vi "LcWebView_BarPlot_Example.vi"() -> ()   [LabVIEW 2019, in "LcWebView.lvclass"]
doc: "Inject javascript arguments"
uses:
  LcWebView.lvclass
  ctrls/PlotType.ctl
  ctrls/BarPlotOption.ctl
  Program Files/National Instruments/LabVIEW 2020/user.lib/_LabVIEWCommon/LcHTMLPlot/HTMLPlot_class/Controls/LegendPosition.ctl
  Program Files/National Instruments/LabVIEW 2020/user.lib/_LabVIEWCommon/LcHTMLPlot/HTMLPlot_class/HTMLPlot.lvclass
  ctrls/GenericPlotOption.ctl
  C:/Projects/WebView2/LcWebView/data/Microsoft.Web.WebView2.WinForms.dll
panel:
  out "BrowserProcessId":u32
  out "Source Change":string
  out "Status Message":string
  in  "stop":bool
  in  "Web":refnum<k24>(container)
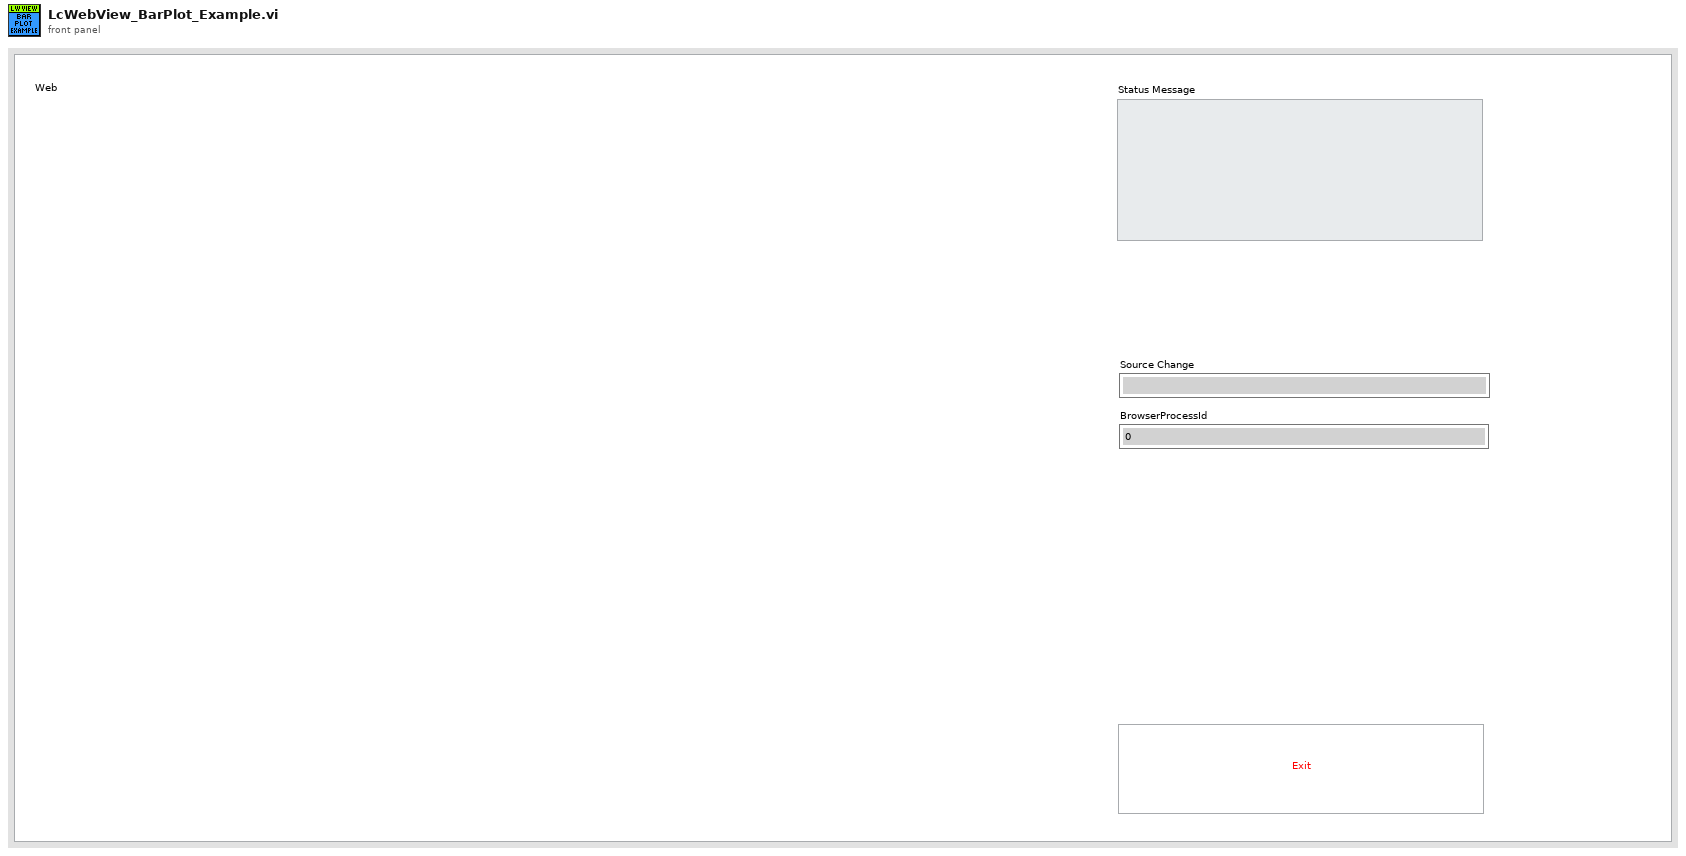
[diagram p1: front panel]
types:
  T1 = typedef "LcWebView.lvclass/PlotType.ctl" = enum16{"bar", "line", "pie"}
  T2 = typedef "LcWebView.lvclass/GenericPlotOption.ctl" = cluster{"GraphTitle":string, "LegendDisplay":bool, "LegendPosition":T3}
  T3 = typedef "HTMLPlot.lvclass/LegendPosition.ctl" = enum16{"top", "right", "left", "bottom"}
  T4 = typedef "LcWebView.lvclass/BarPlotOption.ctl" = cluster{"xLabel":string, "yLabel":string, "DisplayXLabel":bool, "DisplayYLabel":bool, "Stacked":bool}
  T5 = typedef "LcWebView.lvclass/WebViewDynamicEvents.ctl" = cluster{"Event Registration Ref":refnum<event-registration>, "Source event":refnum<user-event>}
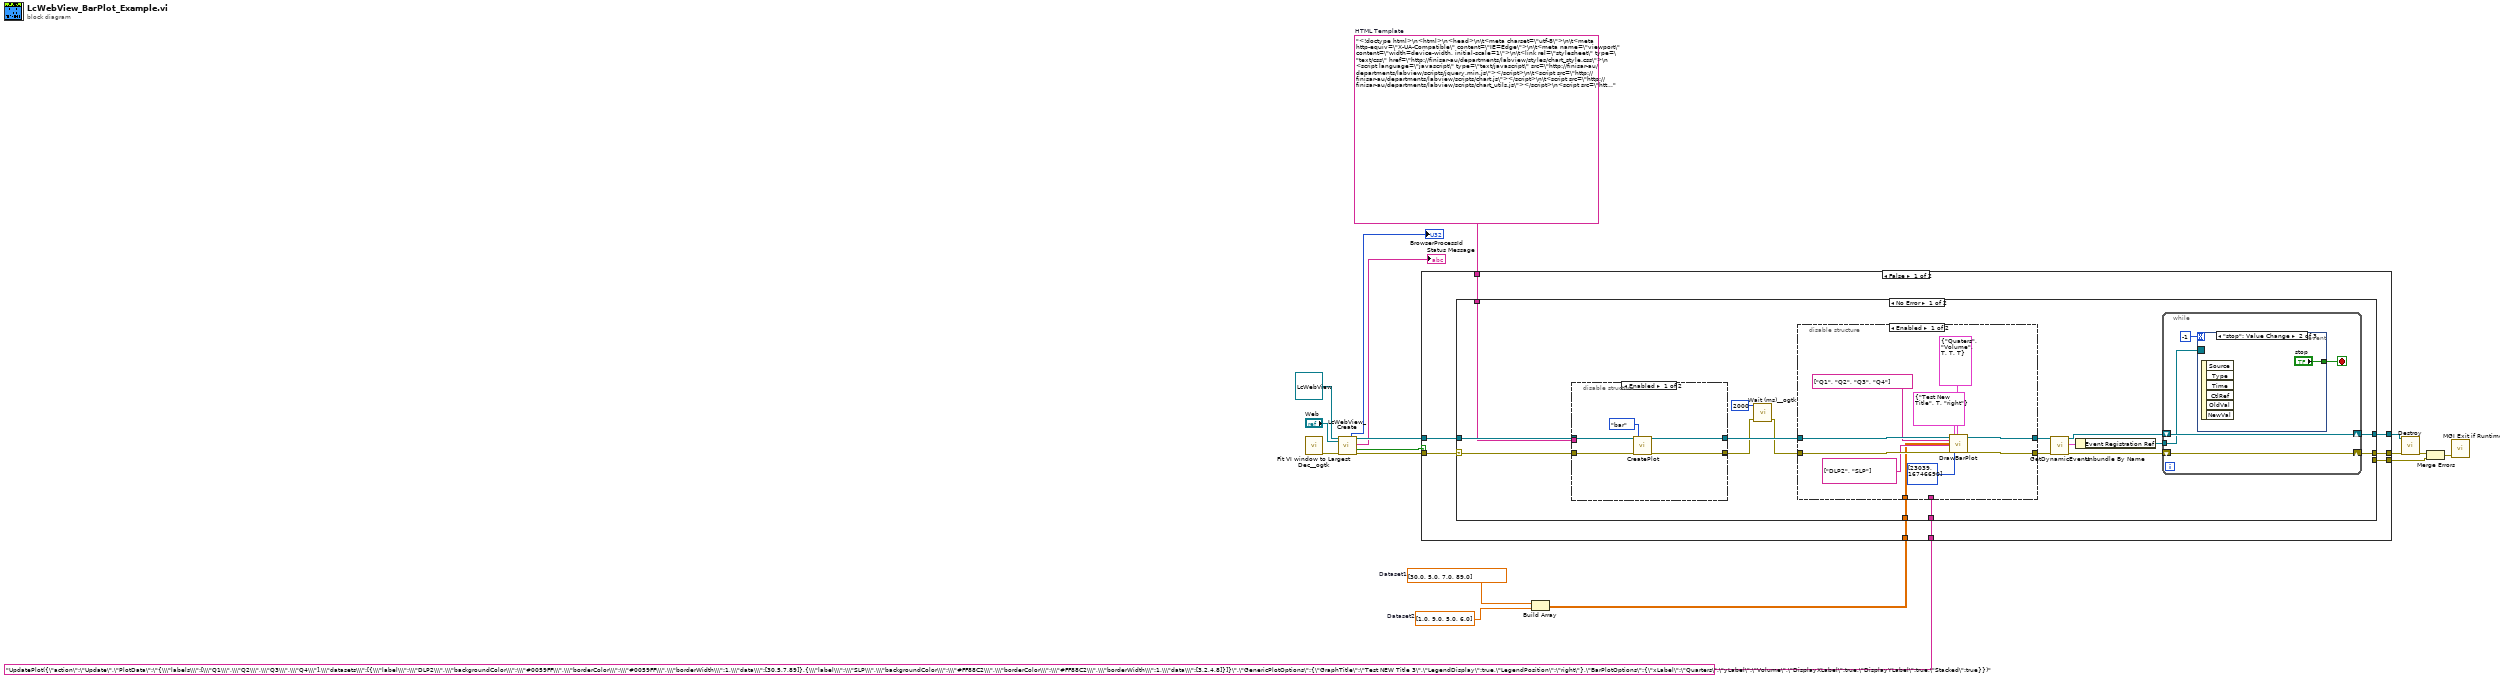
[diagram p0: block diagram]
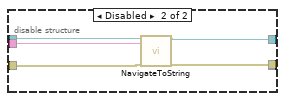
[diagram p2: hidden frame]
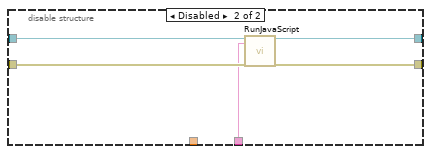
[diagram p3: hidden frame]
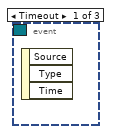
[diagram p4: hidden frame]
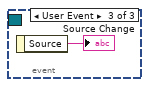
[diagram p5: hidden frame]
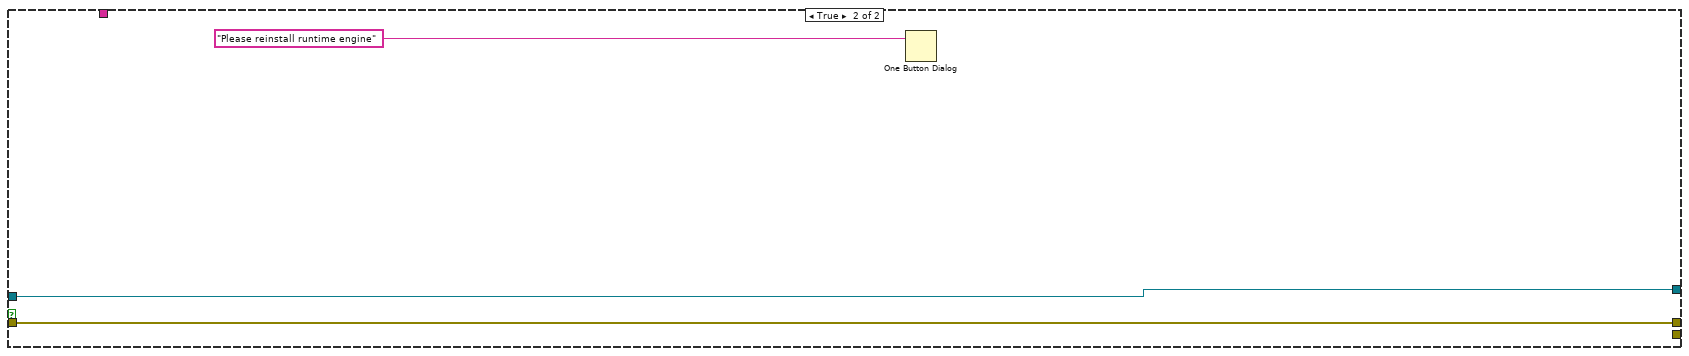
[diagram p7: hidden frame]
diagram:
  w1 = "<!doctype html>\n<html>\n<head>\n\t<meta charset=\"utf-8\">\n\t<meta http-equiv=\"X-UA-Compatible\" content=\"IE=Edge\">\n\t<meta name=\"viewport\" content=\"width=device-width, initial-scale=1\">\n\t<link rel=\"stylesheet\" type=\"text/css\" href=\"http://finisar-au/departments/labview/styles/chart_style.css\">\n <script language=\"javascript\" type=\"text/javascript\" src=\"http://finisar-au/departments/labview/scripts/jquery.min.js\"></script>\n\t<script src=\"http://finisar-au/departments/labview/scripts/chart.js\"></script>\n\t<script src=\"http://finisar-au/departments/labview/scripts/chart_utils.js\"></script>\n<script src=\"http://finisar-au/departments/labview/scripts/json2.js\"></script>\n    <script src=\"http://finisar-au/departments/labview/scripts/jquery(v1.11.3).min.js\"></script>\n    <style>\n    \t#container{\n            width:95vm;\n            height:95vh;\n            }\n        #canvas {\n\t\t-moz-user-select: none;\n\t\t-webkit-user-select: none;\n\t\t-ms-user-select: none;  \n\t   }\n\t    </style>\n</head>\n\n<body>\n<div id=\"container\">\n\t\t<canvas id=\"canvas\"></canvas>\n\t</div>\n\t<script type=\"text/javascript\">\n//---colour helper\nvar color = Chart.helpers.color;\nvar plotData ={}  \n\n // summarise config here --------------------------                   \n        var config = {\n\n// **************** PLOT TYPE***************************\n\t\t\ttype: 'bar',\n\n\t\t\tdata: plotData,\n//\t\t\t **************** PLOT OPTIONS : THIS PART WILL BE PLOT TYPE DEPENDENT***************************\noptions: \n{\nresponsive: true,\nmaintainAspectRatio: false,\n\t\t\t\tanimation: {\n\t\t\t\t\tanimateScale: true,\n\t\t\t\t\tanimateRotate: true\n\t\t\t\t},\nlegend: {\ndisplay:false,\t\t\t\t\t\t\nposition: 'right'\n\t\t\t\t\t},\ntitle: {\n\t\t\t\t\t\tdisplay:true,\n\t\t\t\t\t\ttext: 'INPUT'\n\t\t\t\t\t},  \n//*************************  ADDITIONAL OPTIONS   ***********************\n\t\t\t\tscales: {\n\t\t\t\t\txAxes: [{\n\t\t\t\t\t\t\tscaleLabel: {\n\t\t\t\t\t\t\tdisplay: true,\n\t\t\t\t\t\t\tlabelString: 'INPUT',\n       stacked:true\n\t\t\t\t\t\t}\n\t\t\t\t\t}],\n\t\t\t\t\tyAxes: [{\n\tticks: {\n\t\t\t\t\t\t\tmin: 0\n\t\t\t\t\t\t\t\t\t\t\t\t\t},\n\t\t\t\t\t\tscaleLabel: {\n\t\t\t\t\t\t\tdisplay: true,\n\t\t\t\t\t\t\tlabelString: 'INPUT',\n       stacked:true\n       \t\t\t\t\t\t}\n\t\t\t\t\t}]\n\t\t\t\t},\ntooltips: {\nenabled: true}\t\n}\n\t\t};\n\n// run plot function here -------------------------- \nwindow.onload = function() {\n\t  var ctx = document.getElementById('canvas').getContext('2d');\n\t\t\twindow.myChart = new Chart(ctx, config); \n};\n\nfunction UpdatePlot(data) {        \n    var myData = JSON.parse(data.PlotData);\n    config.data=myData;\n\tconfig.options.legend.display= data.GenericPlotOptions.LegendDisplay;\n\tconfig.options.legend.position=data.GenericPlotOptions.LegendPosition;            \n\tconfig.options.title.text=data.GenericPlotOptions.GraphTitle;\n\n//*************************  ADDITIONAL OPTIONS UPDATE ***********************\n\tconfig.options.scales.yAxes[0].stacked=data.BarPlotOptions.Stacked;\n\tconfig.options.scales.xAxes[0].stacked=data.BarPlotOptions.Stacked;\n\tconfig.options.scales.xAxes[0].scaleLabel.labelString=data.BarPlotOptions.xLabel;\n\tconfig.options.scales.yAxes[0].scaleLabel.labelString=data.BarPlotOptions.yLabel;\n\tconfig.options.scales.yAxes[0].scaleLabel.display=data.BarPlotOptions.DisplayYLabel;\n\tconfig.options.scales.xAxes[0].scaleLabel.display=data.BarPlotOptions.DisplayXLabel;\n\n//*************************  UPDATE PLOT ***********************\n\twindow.myChart.update();\n}\n\t</script>\n</body>\n</html>"  # HTML Template
  w5 = dbl[] [1.0, 9.0, 5.0, 6.0]  # Dataset2
  w4 = dbl[] [30.0, 5.0, 7.0, 89.0]  # Dataset1
  n1 = call "Fit VI window to Largest Dec__ogtk.vi"() -> ("error out"=w8:errorcluster)  [unwired: 6 in, 1 out]
  n2 = call "LcWebView_Create.vi"("reference in"=refnum<class "LcWebView.lvclass"> refnum, "Webview container"="Web", "Error In"=w8) -> ("BrowserProcessId"=→"BrowserProcessId":u32, "reference out"=w16:refnum<class "LcWebView.lvclass">, "Status Message"=→"Status Message":string, "Reinstall Runtime"=w9:bool, "Error Out"=w15:errorcluster)  [unwired: 9 in, 3 out]
  n3 = Build Array(w4, w5) -> (w3:dbl[][])
  n4 = case shown="False" w9 {
    tunnel: w16 -> [w26 w80]
    tunnel: w15 -> [w25 w79]
    tunnel: [w24 w80] -> w14
    tunnel: [w22 w79] -> w13
    tunnel: [w23 _] -> w10
    tunnel: w3 -> [w21 _]
    tunnel: "UpdatePlot({\"action\":\"Update\",\"PlotData\":\"{\\\"labels\\\":[\\\"Q1\\\",\\\"Q2\\\",\\\"Q3\\\",\\\"Q4\\\"],\\\"datasets\\\":[{\\\"label\\\":\\\"DLP2\\\",\\\"backgroundColor\\\":\\\"#0059FF\\\",\\\"borderColor\\\":\\\"#0059FF\\\",\\\"borderWidth\\\":1,\\\"data\\\":[30,5,7,89]},{\\\"label\\\":\\\"SLP\\\",\\\"backgroundColor\\\":\\\"#FF88C2\\\",\\\"borderColor\\\":\\\"#FF88C2\\\",\\\"borderWidth\\\":1,\\\"data\\\":[3,2,4,8]}]}\",\"GenericPlotOptions\":{\"GraphTitle\":\"Test NEW Title 3\",\"LegendDisplay\":true,\"LegendPosition\":\"right\"},\"BarPlotOptions\":{\"xLabel\":\"Quarters\",\"yLabel\":\"Volume\",\"DisplayXLabel\":true,\"DisplayYLabel\":true,\"Stacked\":true}})" ("Java Script Function") -> [w20 _]
    tunnel: w1 -> [w19 _]
    frame False {
      n5 = case shown="No Error" w25 {
        selector: w25 -> [w40 w76]
        tunnel: w26 -> [w41 w77]
        tunnel: [w37 w77] -> w24
        tunnel: [w43 _] -> w22
        tunnel: [_ w76] -> w23
        tunnel: w21 -> [w32 _]
        tunnel: w20 -> [w31 _]
        tunnel: w19 -> [w30 _]
        frame No Error {
          n6 = disable-structure shown="Enabled" {
            disable-tunnel: w41 -> [w48 w53]
            disable-tunnel: w40 -> [w47 w50]
            disable-tunnel: [w45 _] -> w29
            disable-tunnel: [w44 w52] -> w33
            disable-tunnel: [_ w51] -> _
            disable-tunnel: w30 -> [_ w49]
            frame Enabled {
              n7 = call-dynamic "CreatePlot.vi"("reference in"=w48, "Error In"=w47, "PlotType"=PlotType."bar") -> ("reference out"=w44:refnum<class "LcWebView.lvclass">, "Error Out"=w45:errorcluster)  [unwired: 15 in]
            }
            frame Disabled {
              n8 = call-dynamic "NavigateToString.vi"("reference in"=w53, "HTML Content"=w49, "Error In"=w50) -> ("reference out"=w52:refnum<class "LcWebView.lvclass">, "Error Out"=w51:errorcluster)  [unwired: 14 in, 1 out]
            }
          }
          n9 = call "Wait (ms)__ogtk.vi"("error in (no error)"=w29, "milliseconds to wait"=u32 2000) -> ("error out"=w28:errorcluster)  [unwired: 8 in, 1 out]
          n10 = disable-structure shown="Enabled" {
            disable-tunnel: [w63 w67] -> w35
            disable-tunnel: [w62 w66] -> w34
            disable-tunnel: w28 -> [w61 w65]
            disable-tunnel: w33 -> [w60 w68]
            disable-tunnel: w32 -> [w54 _]
            disable-tunnel: w31 -> [_ w64]
            frame Enabled {
              n11 = call-dynamic "DrawBarPlot.vi"("reference in"=w60, "XLabels"=string[] ["Q1", "Q2", "Q3", "Q4"], "BarPlot.Dataset"=w54, "BarPlot.DatasetLabels"=string[] ["DLP2", "SLP"] ("DatasetLabels"), "Error In"=w61, "GenericPlotOptions"=T2 {"GraphTitle"="Test New Title", "LegendDisplay"=TRUE, "LegendPosition"=enum."right"}, "BarPlot.PlotColours"=u32[] [23039, 16746690] ("PlotColours"), "BarPlotOptions"=T4 {"xLabel"="Quaters", "yLabel"="Volume", "DisplayXLabel"=TRUE, "DisplayYLabel"=TRUE, "Stacked"=TRUE}) -> ("reference out"=w63:refnum<class "LcWebView.lvclass">, "Error Out"=w62:errorcluster)  [unwired: 10 in]
            }
            frame Disabled {
              n12 = call-dynamic "RunJavaScript.vi"("reference in"=w68, "Java Script Function"=w64, "Error In"=w65) -> ("reference out"=w67:refnum<class "LcWebView.lvclass">, "Error Out"=w66:errorcluster)  [unwired: 13 in, 2 out]
            }
          }
          n13 = call-dynamic "GetDynamicEvents.vi"("reference in"=w35, "Error In"=w34) -> ("reference out"=w38:refnum<class "LcWebView.lvclass">, "DynamicEvents"=w36:T5, "Error Out"=w39:errorcluster)  [unwired: 15 in]
          n14 = Unbundle By Name(w36) -> ("Event Registration Ref"=w42:refnum<event-registration>)
          n15 = while {
            shift-right: [w73] -> w37
            shift-left: w38 -> [w73]
            shift-right: [w72] -> w43
            shift-left: w39 -> [w72]
            tunnel: w42 -> [w69]
            stop <- w70 stop-if-true
            n16 = event shown="[1] \"stop\": Value Change" {
              selector: w69 -> [_ _ _]
              dyn-events: _ -> [_ _ _]
              timeout: -1 -> [_ _ _]
              tunnel: [_ "stop" _] -> w70
              event Timeout {
                n17 = event-data() -> ()  [unwired: 1 in, 3 out]
              }
              event "stop": Value Change {
                n18 = event-data() -> ()  [unwired: 1 in, 6 out]
              }
              event User Event {
                n19 = event-data() -> ("Source"=→"Source Change":string)  [unwired: 1 in]
              }
            }
          }
        }
        frame Error {
        }
      }
    }
    frame True {
      n20 = One Button Dialog(message="Please reinstall runtime engine") -> ()  [unwired: 1 in, 1 out]
    }
  }
  n21 = call-dynamic "Destroy.vi"("reference in"=w14, "Error In"=w13) -> ("Error Out"=w12:errorcluster)  [unwired: 16 in, 1 out]
  n22 = Merge Errors(w12, w10) -> (w7:errorcluster)
  n23 = call "MGI Exit if Runtime.vi"("Error In (Dependency Only)"=w7) -> ()  [unwired: 11 in]
